vi "Globals.vi"() -> ()   [LabVIEW 2015, in "AMC.lvlib"]
uses:
  AMC.lvlib
panel:
  in  "UDPPortsToTry":i32=250
  in  "Ack Message Name":string="AMC_Ack"
  in  "Default UDP Port":u16=54321
  in  "Dispatcher Process Name":string="AMC_Dispatch"
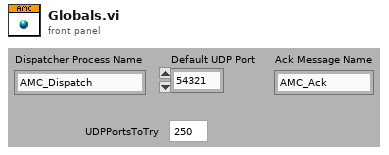
[diagram p1: front panel]
diagram:
